vi "WriteRead Data.vi"(7 "SPI Connection":refnum<class "SPI Connection.lvclass">, 8 "error in (no error)":errorcluster, 10 "Write Data":string) -> (0 "error out":errorcluster, 1 "Read Data":string)   [LabVIEW 2024, in "CTI.lvlib" / "SPI Connection.lvclass"]
uses:
  SPI Connection.lvclass
  SPI Connection.lvclass/SPI Connection.ctl
  Session/Session.lvclass
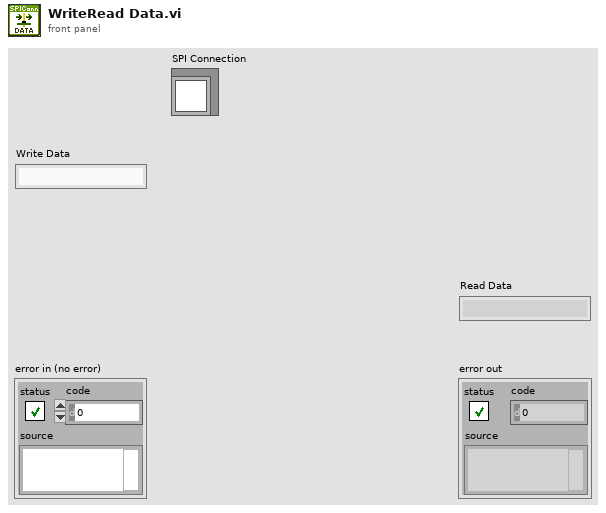
[diagram p1: front panel]
types:
  T1 = typedef "CTI.lvlib/SPI Number.ctl" = i8
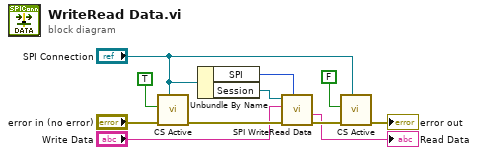
[diagram p0: block diagram]
diagram:
  n1 = call "CS Active.vi"("SPI Connection"="SPI Connection", "error in (no error)"="error in (no error)", "CS Active"=TRUE) -> ("error out"=w10:errorcluster)  [unwired: 8 in]
  n2 = Unbundle By Name("SPI Connection") -> ("SPI"=w9:T1, "Session"=w1:refnum<class "Session.lvclass">)
  n3 = call "SPI WriteRead Data.vi"("SPI #"=w9, "error in (no error)"=w10, "Write Data"="Write Data", "Session in"=w1) -> ("error out"=w11:errorcluster, "Read Data"=→"Read Data":string)  [unwired: 5 in, 1 out]
  n4 = call "CS Active.vi"("SPI Connection"="SPI Connection", "error in (no error)"=w11, "CS Active"=FALSE) -> ("error out"=→"error out":errorcluster)  [unwired: 8 in]
